vi "moveMotorREL.vi"(8 "error in (no error)":errorcluster, 9 "Axis":enum16{"X", "Y"}(ring), 10 "L (mm)":dbl, 11 "VISA Refnum in":refnum<visa-resource-name>) -> (0 "error out":errorcluster, 3 "VISA Refnum out":refnum<visa-resource-name>)   [LabVIEW 2014]
doc: "Newport Motion Controler\nThis subVI move motor relative postion \n\nAndré Romero - 2020\nandretec@ifsc.usp.br"
uses:
  Global Motor Axis.vi
  <userlib>/Newport ESP301/Newport ESP301.lvlib
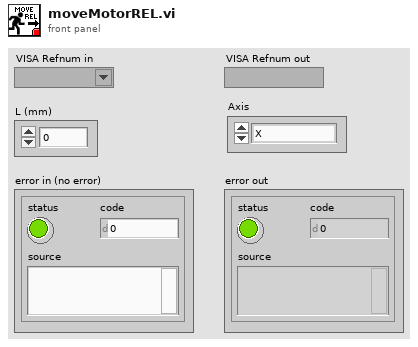
[diagram p1: front panel]
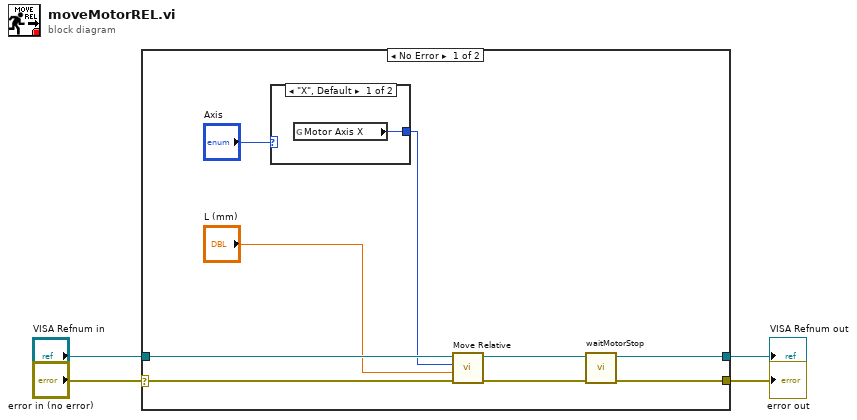
[diagram p0: block diagram]
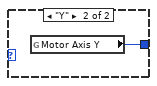
[diagram p2: hidden frame]
diagram:
  n1 = case shown="No Error" "error in (no error)" {
    selector: "error in (no error)" -> [w5 w16]
    tunnel: "VISA Refnum in" -> [w13 w17]
    tunnel: [w12 w16] -> w3
    tunnel: [w11 w17] -> w2
    frame No Error {
      n2 = case shown="\"X\", Default" "Axis" {
        tunnel: [w14 w15] -> w6
        frame "X", Default {
          n3 = global read "Global Motor Axis.vi" "Motor Axis X"() -> (w14:i32)
        }
        frame "Y" {
          n4 = global read "Global Motor Axis.vi" "Motor Axis Y"() -> (w15:i32)
        }
      }
      n5 = call <userlib>:"Move Relative.vi"("error in (no error)"=w5, "Position (0 units)"="L (mm)", "Axis (1)"=w6, "VISA resource name"=w13) -> ("error out"=w9:errorcluster, "VISA resource name out"=w8:refnum<visa-resource-name>)  [unwired: 2 in]
      n6 = call "waitMotorStop.vi"("error in (no error)"=w9, "VISA Refnum in"=w8) -> ("error out"=w12:errorcluster, "VISA Refnum out"=w11:refnum<visa-resource-name>)  [unwired: 8 in]
    }
    frame Error {
    }
  }
  "error out" <- w3
  "VISA Refnum out" <- w2
